vi "commandDisable.vi"(8 "error in (no error)":errorcluster, 10 "CommandDisable in":T1, 11 "M1M3SAL in":refnum<class "M1M3SAL.lvclass">) -> (0 "error out":errorcluster, 2 "CommandDisable out":T1, 3 "M1M3SAL out":refnum<class "M1M3SAL.lvclass">)   [LabVIEW 2016, in "M1M3Communicator.lvlib" / "M1M3SAL.lvclass"]
uses:
  M1M3SAL.lvclass
  Topics/CommandDisable.ctl
  Topics/CommandId.ctl
  DataTypes/MessageHeader.ctl
  DataTypes/MessageTypes.ctl
  DataTypes/MessageTopics.ctl
  Common_RT_Utilities/U8ArrayBuilderAutoIndexing/U8ArrayBuilderAutoIndexing.lvclass
  M1M3Communicator.lvlib
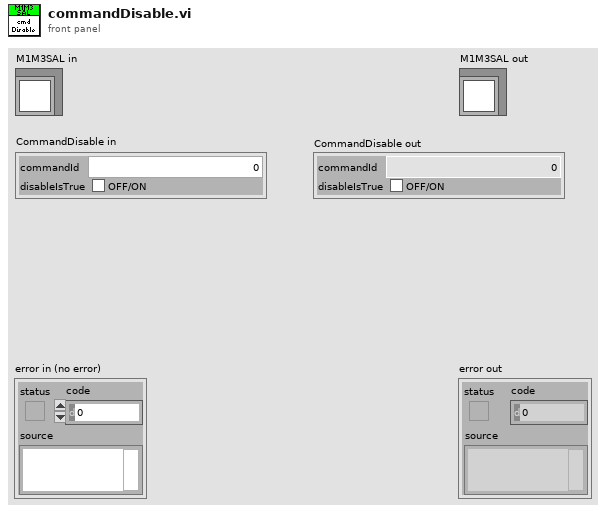
[diagram p1: front panel]
types:
  T1 = typedef "M1M3Communicator.lvlib/CommandDisable.ctl" = cluster{"commandId":T2, "disableIsTrue":bool}
  T2 = typedef "M1M3Communicator.lvlib/CommandId.ctl" = i32
  T3 = typedef "M1M3Communicator.lvlib/MessageHeader.ctl" = cluster{"Type":T4, "Topic":T5, "Size":i32}
  T4 = typedef "M1M3Communicator.lvlib/MessageTypes.ctl" = enum8{"None", "PutSample", "GetNextSample", "LogEvent", "GetEvent", "IssueCommand", "CommandId", "WaitForCompletion", "AcceptCommand", "AckCommand"}
  T5 = typedef "M1M3Communicator.lvlib/MessageTopics.ctl" = enum8{"None", "Start", "Enable", "Disable", "Standby", "AppliedSettingsMatchStart", "ErrorCode", "SettingVersions", "SummaryState", "DetailedState", "Exit"}
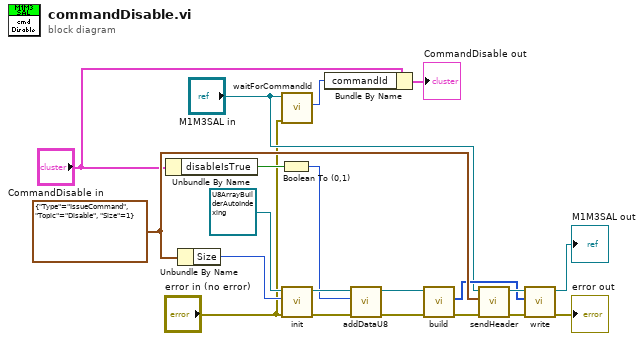
[diagram p0: block diagram]
diagram:
  w19 = T3 {"Type"=enum."IssueCommand", "Topic"=enum."Disable", "Size"=1} ("MessageHeader")
  n1 = Unbundle By Name("CommandDisable in") -> ("disableIsTrue"=w15:bool)
  n2 = Unbundle By Name(w19) -> ("Size"=w18:i32)
  n3 = Boolean To (0,1)(Boolean=w15) -> (0, 1=w16:i16)
  n4 = call "waitForCommandId.vi"("error in (no error)"="error in (no error)", "M1M3SAL in"="M1M3SAL in") -> ("CommandId"=w6:T2)  [unwired: 7 in, 2 out]
  n5 = call "init.vi"("error in (no error)"="error in (no error)", "Size"=w18, "U8ArrayBuilderAutoIndexing in"=refnum<class "U8ArrayBuilderAutoIndexing.lvclass"> refnum ("RTUtilities.lvlib:U8ArrayBuilderAutoIndexing.lvclass")) -> ("error out"=w11:errorcluster, "U8ArrayBuilderAutoIndexing out"=w17:refnum<class "U8ArrayBuilderAutoIndexing.lvclass">)  [unwired: 7 in]
  n6 = Bundle By Name(cluster="CommandDisable in", "commandId"=w6) -> (→"CommandDisable out":T1)
  n7 = call "addDataU8.vi"("error in (no error)"=w11, "Data"=w16, "U8ArrayBuilderAutoIndexing in"=w17) -> ("error out"=w10:errorcluster, "U8ArrayBuilderAutoIndexing out"=w14:refnum<class "U8ArrayBuilderAutoIndexing.lvclass">)  [unwired: 7 in]
  n8 = call "build.vi"("error in (no error)"=w10, "U8ArrayBuilderAutoIndexing in"=w14) -> ("error out"=w9:errorcluster, "Array"=w12:u8[])  [unwired: 7 in, 1 out]
  n9 = call "sendHeader.vi"("error in (no error)"=w9, "MessageHeader"=w19, "M1M3SAL in"="M1M3SAL in") -> ("error out"=w8:errorcluster, "M1M3SAL out"=w13:refnum<class "M1M3SAL.lvclass">)  [unwired: 7 in]
  n10 = call "write.vi"("error in (no error)"=w8, "Data"=w12, "M1M3SAL in"=w13) -> ("error out"=→"error out":errorcluster, "M1M3SAL out"=→"M1M3SAL out":refnum<class "M1M3SAL.lvclass">)  [unwired: 7 in]
